vi "Read message.vi"(8 "error in":errorcluster, 9 "timeout ms (25000)":i32=25000, 11 "Connection Info":T1) -> (0 "error out":errorcluster, 1 "Messsage value":string, 2 "Message name":string, 3 "Connection Info out":T1)   [LabVIEW 2021]
uses:
  Connection Info.ctl
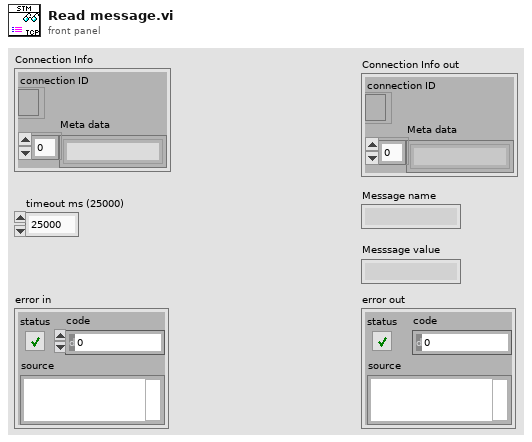
[diagram p1: front panel]
types:
  T1 = typedef "Connection Info.ctl" = cluster{"connection ID":refnum<k5>, "Meta data":string[]}
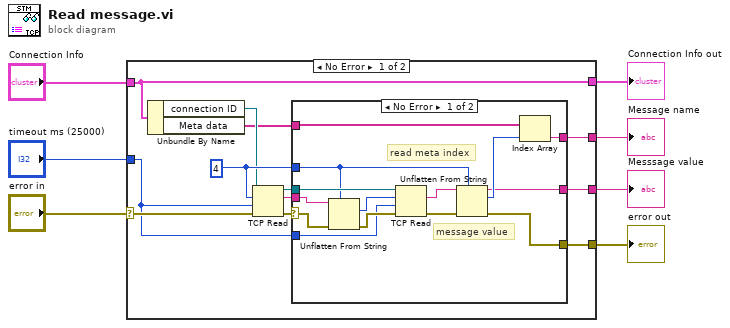
[diagram p0: block diagram]
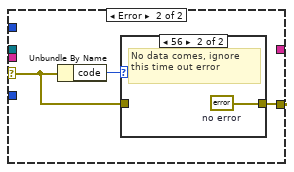
[diagram p2: hidden frame]
diagram:
  n1 = case shown="No Error" "error in" {
    selector: "error in" -> [w19 w40]
    tunnel: "Connection Info" -> [w9 w39]
    tunnel: "timeout ms (25000)" -> [w10 _]
    tunnel: [w12 _] -> w5
    tunnel: [w11 _] -> w4
    tunnel: [w8 w40] -> w3
    tunnel: [w9 w39] -> w1
    frame No Error {
      w16 = 4 ("bytes to read")
      n2 = Unbundle By Name(w9) -> ("connection ID"=w15:refnum<k5>, "Meta data"=w13:string[])
      n3 = TCP Read(connection ID=w15, bytes to read=w16, error in (no error)=w19, 9:w10) -> (connection ID out=w14:refnum<k5>, data out=w17:string, error out=w18:errorcluster)  [unwired: 1 in]
      n4 = case shown="No Error" w18 {
        selector: w18 -> [w32 w36]
        tunnel: w17 -> [w33 _]
        tunnel: w16 -> [w28 _]
        tunnel: w14 -> [w30 _]
        tunnel: w13 -> [w24 _]
        tunnel: [w23 _] -> w12
        tunnel: [w21 _] -> w11
        tunnel: [w22 w35] -> w8
        tunnel: w10 -> [w20 _]
        frame No Error {
          # "message value"
          # "read meta index"
          n5 = Unflatten From String(type=w28, binary string=w33, error in (no error)=w32) -> (value=w31:i32, error out=w29:errorcluster)  [unwired: 2 in, 1 out]
          n6 = TCP Read(connection ID=w30, bytes to read=w31, error in (no error)=w29, 9:w20) -> (data out=w27:string, error out=w26:errorcluster)  [unwired: 1 in, 1 out]
          n7 = Unflatten From String(type=w28, binary string=w27, error in (no error)=w26) -> (rest of the binary string=w21:string, value=w25:i32, error out=w22:errorcluster)  [unwired: 2 in]
          n8 = Index Array(array=w24, index=w25) -> (element=w23:string)
        }
        frame Error {
          n9 = Unbundle By Name(w36) -> ("code"=w34:i32)
          n10 = case shown="56" w34 {
            tunnel: w36 -> [w37 _]
            tunnel: [w37 w38] -> w35
            frame 0, Default {
            }
            frame 56 {
              w38 = errorcluster {"status"=FALSE, "code"=0, "source"=""}  # no error
              # "No data comes, ignore this time out error"
            }
          }
        }
      }
    }
    frame Error {
    }
  }
  "Message name" <- w5
  "Messsage value" <- w4
  "error out" <- w3
  "Connection Info out" <- w1
